vi "GEA2 Serial Wait for Bus Idle.vi"(8 "Error In":errorcluster, 10 "Idle Time":u32, 11 "ComPort":refnum<visa-resource-name>) -> (0 "error out":errorcluster, 2 "Bytes at Port":u32)   [LabVIEW 2014]
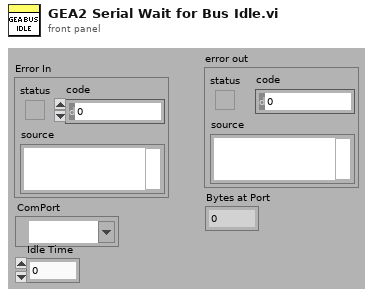
[diagram p1: front panel]
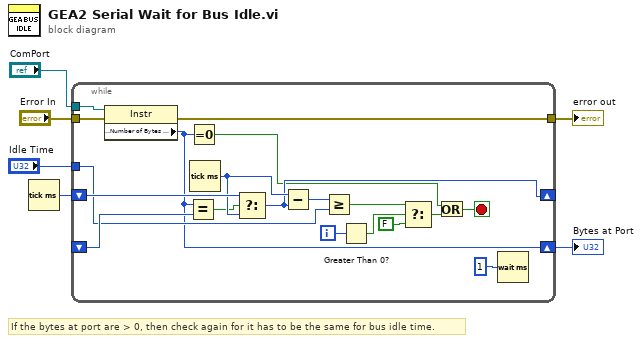
[diagram p0: block diagram]
diagram:
  # "If the bytes at port are > 0, then check again for it has to be the same for bus idle time."
  n1 = Tick Count (ms)() -> (millisecond timer value=w3:u32)
  n2 = while {
    tunnel: "Error In" -> [w25]
    tunnel: [w24] -> w5
    tunnel: "ComPort" -> [w23]
    shift-right: [w8] -> w1
    shift-left: _ -> [w22]
    shift-right: [w17] -> _
    shift-left: w3 -> [w20]
    tunnel: "Idle Time" -> [w10]
    i -> [w15]
    stop <- w9 stop-if-true
    n3 = property class="Instr"(reference=w23, error in=w25) -> (error out=w24:errorcluster, "Serial Settings:Number of Bytes at Serial Port"=w8:u32)  [unwired: 1 out]
    n4 = Equal?(x=w8, y=w22) -> (x = y?=w16:bool)
    n5 = Equal To 0?(x=w8) -> (x = 0?=w7:bool)
    n6 = Tick Count (ms)() -> (millisecond timer value=w18:u32)
    n7 = Select(t=w20, s=w16, f=w18) -> (s? t:f=w17:u32)
    n8 = Subtract(x=w18, y=w17) -> (x-y=w19:u32)
    n9 = Greater Or Equal?(x=w19, y=w10) -> (x >= y?=w14:bool)
    n10 = Greater Than 0?(x=w15) -> (x > 0?=w13:bool)
    n11 = Select(t=w14, s=w13, f=FALSE) -> (s? t:f=w11:bool)
    n12 = Or(x=w7, y=w11) -> (x .or. y?=w9:bool)
    n13 = Wait (ms)(milliseconds to wait=u32 1) -> ()  [unwired: 1 out]
  }
  "error out" <- w5
  "Bytes at Port" <- w1
